vi "SubVIEW1.vi"() -> ()   [LabVIEW 2020]
panel:
  out "高温泵压力#3":dbl(slide) scale=0.0..10.0
  out "高温泵压力#2":dbl(slide) scale=0.0..10.0
  out "高温泵压力#1":dbl(slide) scale=0.0..10.0
  in  "被试泵流量#3":dbl(slide) scale=0.0..10.0
  out "被试泵流量#2":dbl(slide) scale=0.0..10.0
  out "被试泵流量#1":dbl(slide) scale=0.0..10.0
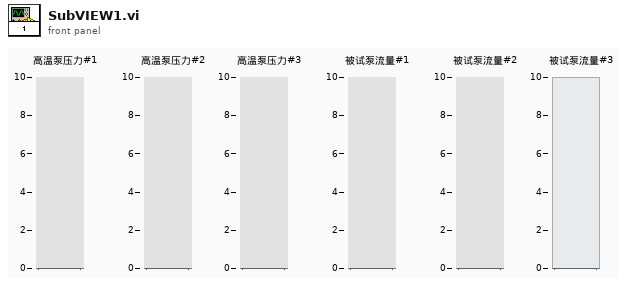
[diagram p1: front panel]
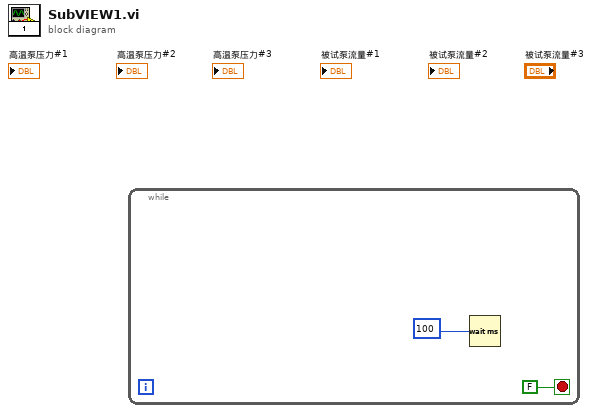
[diagram p0: block diagram]
diagram:
  n1 = while {
    stop <- FALSE stop-if-true
    n2 = Wait (ms)(milliseconds to wait=u32 100 ("millisecond timer value")) -> ()  [unwired: 1 out]
  }
